vi "Integrate.vi"(10 "dt":dbl, 11 "Acceleration":dbl) -> (2 "Displacememt":dbl, 3 "Velocity":dbl)   [LabVIEW 2012]
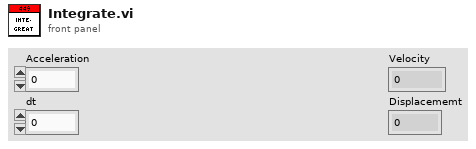
[diagram p1: front panel]
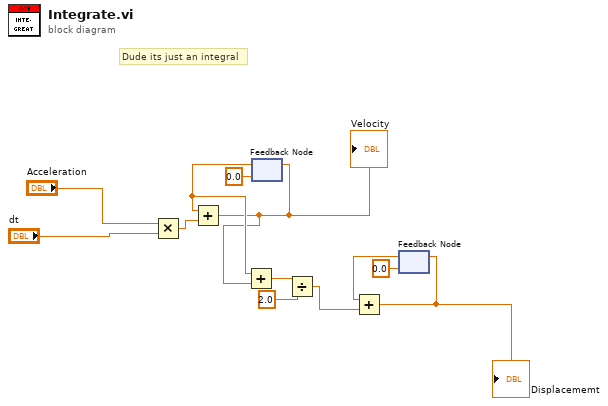
[diagram p0: block diagram]
diagram:
  # "Dude its just an integral"
  n1 = Multiply(x="Acceleration", y="dt") -> (x*y=w12:dbl)
  n2 = feedback #1(0.0) -> (w5:dbl)
  n3 = Add(x=w5, y=w12) -> (x+y=w4:dbl)
  "Velocity" <- w4
  n4 = Add(x=w5, y=w4) -> (x+y=w3:dbl)
  n5 = feedback-in #1(w4) -> ()
  n6 = Divide(x=w3, y=2.0) -> (x/y=w1:dbl)
  n7 = feedback #2(0.0) -> (w8:dbl)
  n8 = Add(x=w8, y=w1) -> (x+y=w9:dbl)
  "Displacememt" <- w9
  n9 = feedback-in #2(w9) -> ()
